vi "Intruder.vi"() -> ()   [LabVIEW 2015]
uses:
  Intruder 2.ctl
panel:
  out "Intrusion Data":timestamp
  in  "stop":bool
  in  "Intrusion Number":i32
  in  "Intruder?":bool
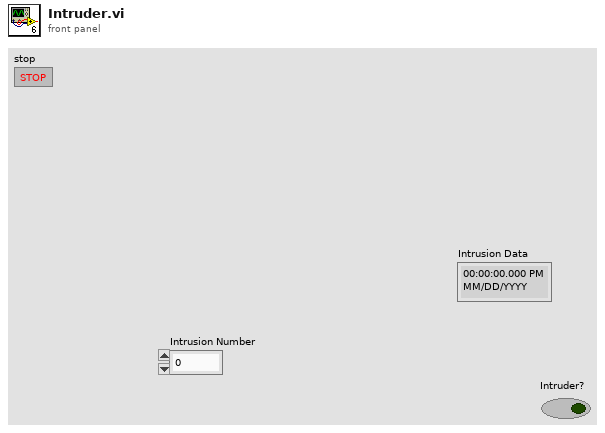
[diagram p1: front panel]
types:
  T1 = typedef "Intruder 2.ctl" = enum16{"Start", "Intruder?", "Log Intrusion"}
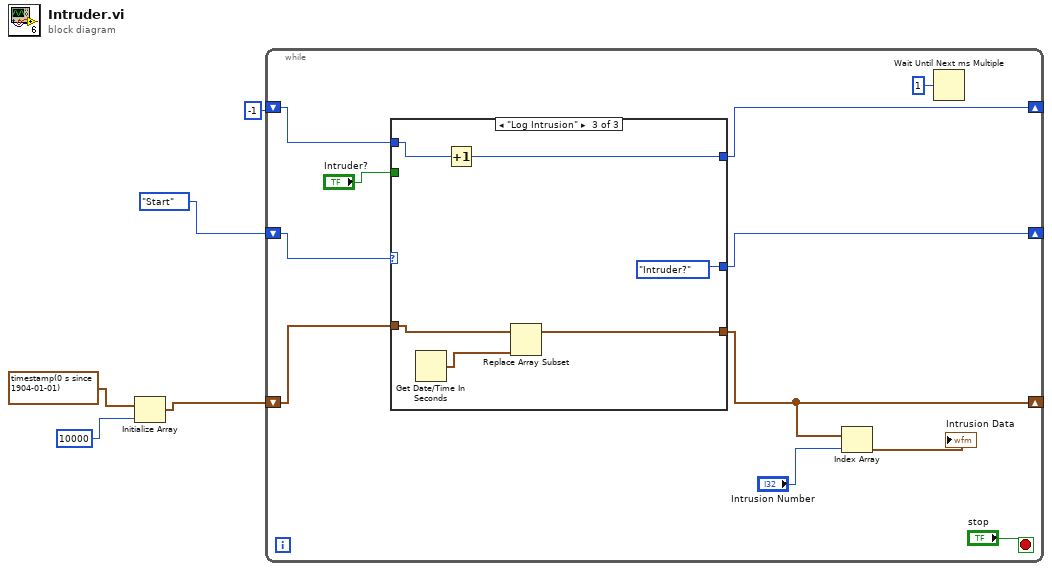
[diagram p0: block diagram]
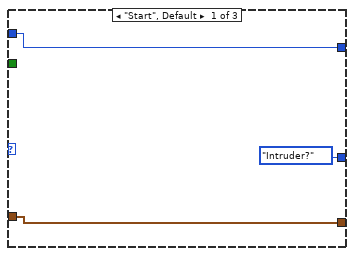
[diagram p2: hidden frame]
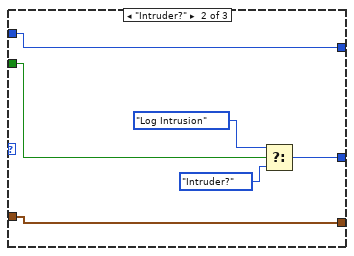
[diagram p3: hidden frame]
diagram:
  n1 = Initialize Array(timestamp(0 s since 1904-01-01), 10000) -> (w1:timestamp[])
  n2 = while {
    shift-right: [w12] -> _
    shift-left: -1 -> [w13]
    shift-right: [w14] -> _
    shift-left: Intruder_2."Start" -> [w15]
    shift-right: [w10] -> _
    shift-left: w1 -> [w11]
    stop <- "stop" stop-if-true
    n3 = case shown="\"Log Intrusion\"" w15 {
      tunnel: "Intruder?" -> [_ w21 _]
      tunnel: [Intruder_2."Intruder?" w20 Intruder_2."Intruder?"] -> w14
      tunnel: w13 -> [w19 w25 w31]
      tunnel: [w19 w25 w30] -> w12
      tunnel: w11 -> [w18 w24 w29]
      tunnel: [w18 w24 w27] -> w10
      frame "Start", Default {
      }
      frame "Intruder?" {
        n4 = Select(t=Intruder_2."Log Intrusion", s=w21, f=Intruder_2."Intruder?") -> (s? t:f=w20:T1)
      }
      frame "Log Intrusion" {
        n5 = Get Date/Time In Seconds() -> (seconds since 1Jan1904=w28:timestamp)
        n6 = Increment(x=w31) -> (x+1=w30:i32)
        n7 = Replace Array Subset(array=w29, new element=w28) -> (w27:timestamp[])  [unwired: 1 in]
      }
    }
    n8 = Index Array(array=w10, index="Intrusion Number") -> (element=→"Intrusion Data":timestamp)
    n9 = Wait Until Next ms Multiple(millisecond multiple=u32 1) -> ()  [unwired: 1 out]
  }
